vi "INA219.vi"() -> ()   [LabVIEW 2018]
uses:
  <vilib>/Instr/_visa.llb/VISA Configure Serial Port (Instr).vi
panel:
  in  "BADC":string
  in  "SADC":string
  in  "PGA":string
  in  "MODE":string
  in  "Enable Termination\nChar (T)":bool=TRUE
  in  "Address":string
  in  "Resistance":string
  in  "VISA resource name":refnum<visa-resource-name>
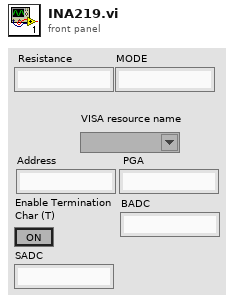
[diagram p1: front panel]
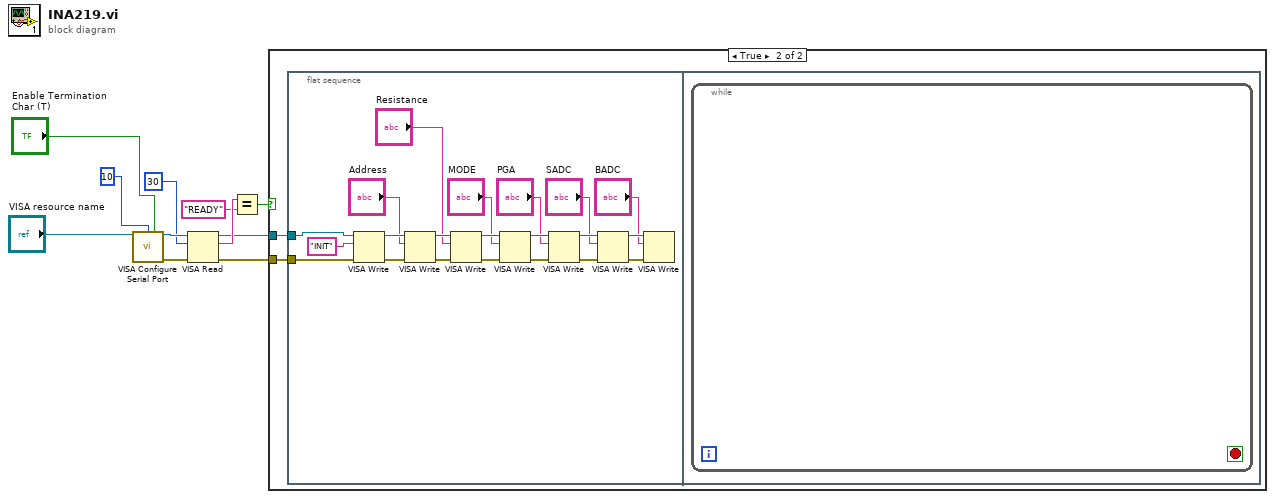
[diagram p0: block diagram]
diagram:
  n1 = call-poly "VISA Configure Serial Port"("VISA resource name"="VISA resource name", "termination char\n(0xA = '\\n' = LF)"=u8 10 ("termination char\n(0xA = '\\n' = LF)"), "Enable Termination\nChar (T)"="Enable Termination\nChar (T)") -> ("VISA resource name out"=w10:refnum<visa-resource-name>, "error out"=w9:errorcluster)  [unwired: 11 in]
  n2 = VISA Read(VISA resource name=w10, byte count=u32 30, error in (no error)=w9) -> (VISA resource name out=w4:refnum<visa-resource-name>, read buffer=w7:string, error out=w3:errorcluster)  [unwired: 1 out]
  n3 = Equal?(x=w7, y="READY") -> (x = y?=w5:bool)
  n4 = case shown="True" w5 {
    tunnel: w4 -> [_ w13]
    tunnel: w3 -> [_ w12]
    frame False {
    }
    frame True {
      n5 = flat-sequence {
        tunnel: w13 -> [w33]
        tunnel: w12 -> [w32]
        frame #0 {
          n6 = VISA Write(VISA resource name=w33, write buffer="INIT", error in (no error)=w32) -> (VISA resource name out=w29:refnum<visa-resource-name>, error out=w31:errorcluster)  [unwired: 1 out]
          n7 = VISA Write(VISA resource name=w29, write buffer="Address", error in (no error)=w31) -> (VISA resource name out=w28:refnum<visa-resource-name>, error out=w30:errorcluster)  [unwired: 1 out]
          n8 = VISA Write(VISA resource name=w28, write buffer="Resistance", error in (no error)=w30) -> (VISA resource name out=w25:refnum<visa-resource-name>, error out=w22:errorcluster)  [unwired: 1 out]
          n9 = VISA Write(VISA resource name=w25, write buffer="MODE", error in (no error)=w22) -> (VISA resource name out=w24:refnum<visa-resource-name>, error out=w21:errorcluster)  [unwired: 1 out]
          n10 = VISA Write(VISA resource name=w24, write buffer="PGA", error in (no error)=w21) -> (VISA resource name out=w23:refnum<visa-resource-name>, error out=w20:errorcluster)  [unwired: 1 out]
          n11 = VISA Write(VISA resource name=w23, write buffer="SADC", error in (no error)=w20) -> (VISA resource name out=w15:refnum<visa-resource-name>, error out=w16:errorcluster)  [unwired: 1 out]
          n12 = VISA Write(VISA resource name=w15, write buffer="BADC", error in (no error)=w16) -> ()  [unwired: 3 out]
        }
        frame #1 {
          n13 = while {
            stop <- _ stop-if-true
          }
        }
      }
    }
  }
